vi "terminate.vi"(8 "error in (no error)":errorcluster, 11 "BalloonNotifier in":refnum<class "BalloonNotifier.lvclass">) -> (0 "error out":errorcluster, 3 "BalloonNotifier out":refnum<class "BalloonNotifier.lvclass">)   [LabVIEW 2010, in "BalloonNotifier.lvclass"]
uses:
  BalloonNotifier.lvclass
  BalloonNotifier.lvclass/BalloonNotifier.ctl
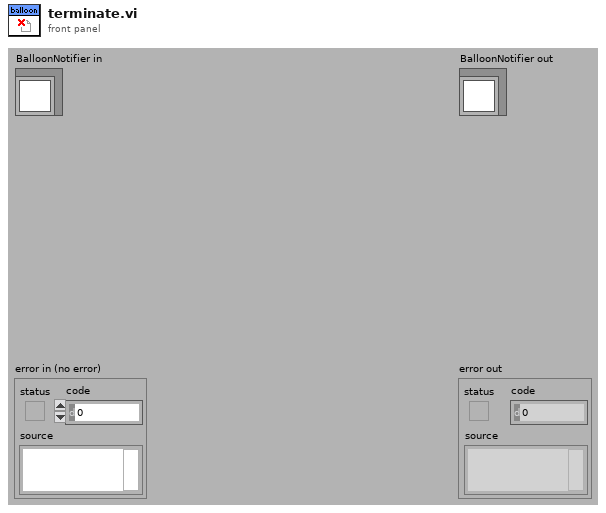
[diagram p1: front panel]
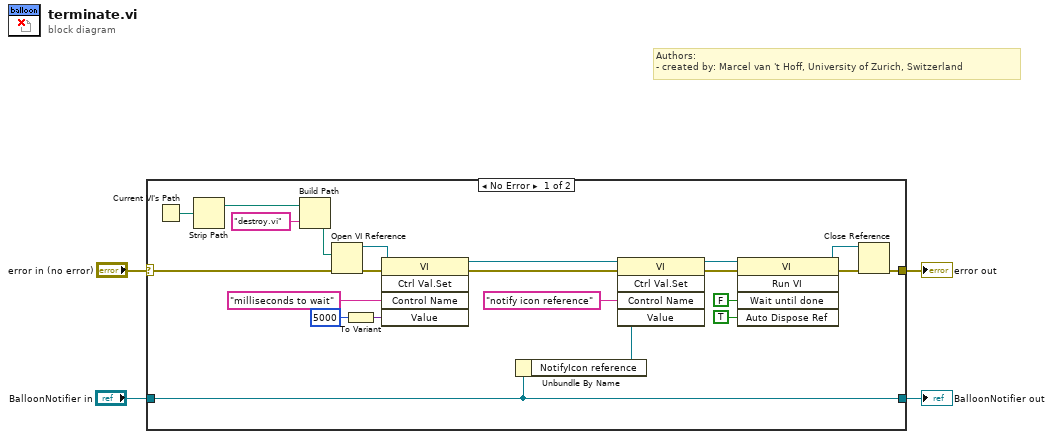
[diagram p0: block diagram]
diagram:
  # "Authors: \n- created by: Marcel van 't Hoff, University of Zurich, Switzerland"
  n1 = case shown="No Error" "error in (no error)" {
    selector: "error in (no error)" -> [w22 w28]
    tunnel: [w5 w28] -> w3
    tunnel: [w20 w27] -> w1
    tunnel: "BalloonNotifier in" -> [w20 w27]
    frame No Error {
      n2 = Current VI's Path() -> (path=w26:path)
      n3 = Strip Path(path=w26) -> (stripped path=w25:path)  [unwired: 1 out]
      n4 = Build Path(base path=w25, name or relative path="destroy.vi") -> (appended path=w23:path)
      n5 = Open VI Reference(vi path=w23, error in (no error)=w22) -> (vi reference=w15:refnum<vi>, error out=w14:errorcluster)  [unwired: 4 in]
      n6 = To Variant(anything=u32 5000) -> (Variant=w17:variant)
      n7 = invoke class="VI" method="Ctrl Val.Set"(reference=w15, error in=w14, "Control Name"="milliseconds to wait", "Value"=w17) -> (reference out=w12:refnum<vi>, error out=w13:errorcluster)  [unwired: 1 in, 3 out]
      n8 = Unbundle By Name(w20) -> ("NotifyIcon reference"=w19:refnum<k24>)
      n9 = invoke class="VI" method="Ctrl Val.Set"(reference=w12, error in=w13, "Control Name"="notify icon reference", "Value"=w19) -> (reference out=w10:refnum<vi>, error out=w11:errorcluster)  [unwired: 1 in, 3 out]
      n10 = invoke class="VI" method="Run VI"(reference=w10, error in=w11, "Wait until done"=FALSE ("Wait Until Done"), "Auto Dispose Ref"=TRUE ("Auto Dispose Reference")) -> (reference out=w7:refnum<vi>, error out=w6:errorcluster)  [unwired: 1 in, 3 out]
      n11 = Close Reference(reference=w7, error in (no error)=w6) -> (error out=w5:errorcluster)
    }
    frame Error {
    }
  }
  "error out" <- w3
  "BalloonNotifier out" <- w1
